vi "Stop Core.vi"(10 "final error code":i32, 11 "Zen Analytics in":refnum<class "Zen Analytics.lvclass">) -> (3 "Zen Analytics out":refnum<class "Zen Analytics.lvclass">)   [LabVIEW 2019, in "Zen Analytics.lvlib" / "Zen Analytics.lvclass"]
doc: "(<B>Filename</B>: Actor Framework.lvlib:Actor.lvclass:Stop Core.vi)\n\nDefines what the actor does before it stops. Use the <B>final error code</B> input to determine whether the actor shut down in response to an error.\n\nBy default, this method does nothing. A descendant class may override it to define behavior, such as shutting down any processes the actor initiated in its override of the Actor Core method."
uses:
  Zen Analytics.lvclass
  <vilib>/ActorFramework/Actor/Actor.lvclass
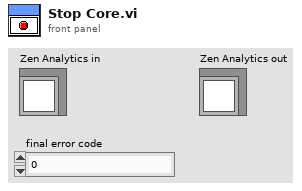
[diagram p1: front panel]
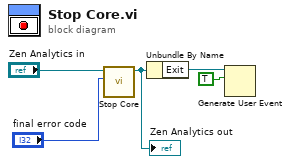
[diagram p0: block diagram]
diagram:
  n1 = call-parent "Stop Core.vi"("final error code"="final error code", "Actor in"="Zen Analytics in") -> ("Actor out"=w3:refnum<class "Zen Analytics.lvclass">)  [unwired: 9 in]
  "Zen Analytics out" <- w3
  n2 = Unbundle By Name(w3) -> ("Exit"=w2:refnum<user-event>)
  n3 = Generate User Event(user event=w2, event data cluster=TRUE ("event data")) -> ()  [unwired: 2 in, 2 out]
